vi "ToTimeStamp.vi"(0 "Time and Date":T1, 7 "Is UTC?":bool=TRUE caption="Is UTC? (T)") -> (4 "Time Stamp":timestamp)   [LabVIEW 2017, in "GPTiming.lvlib"]
doc: "Converts a GPower <B>Time and Date</B> structure into a LabVIEW <B>Time Stamp</B>.\n\nSteen Schmidt\nGPower\n8/5 2016"
uses:
  GPTiming.lvlib
  Date.ctl
  Time.ctl
  TimeAndDate.ctl
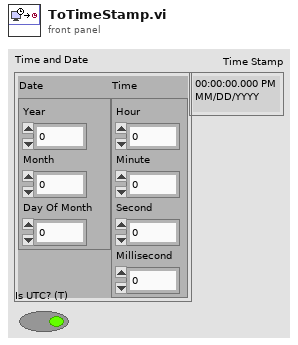
[diagram p1: front panel]
types:
  T1 = typedef "GPTiming.lvlib/TimeAndDate.ctl" = cluster{"Date":T2, "Time":T3}
  T2 = typedef "GPTiming.lvlib/Date.ctl" = cluster{"Year":u16, "Month":u16, "Day Of Month":u16}
  T3 = typedef "GPTiming.lvlib/Time.ctl" = cluster{"Hour":u16, "Minute":u16, "Second":u16, "Millisecond":u16}
  T4 = typedef "LVDateTimeRec.ctl" = cluster{"fractional second":dbl, "second":i32, "minute":i32, "hour":i32, "day of month":i32, "month":i32, "year":i32, "day of week":i32, "day of year":i32, "DST":i32}
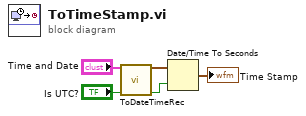
[diagram p0: block diagram]
diagram:
  n1 = call "ToDateTimeRec.vi"("Time and Date"="Time and Date") -> ("Date Time Record"=w3:T4)  [unwired: 14 in]
  n2 = Date/Time To Seconds(1:"Is UTC?", 2:w3) -> (0:→"Time Stamp":timestamp)
